vi "Do Something.vi"(8 "error in (no error)":errorcluster, 10 "Bytes to Read":i32, 11 "Inst.MOTOR in":refnum<class "Inst.MOTOR.lvclass">) -> (0 "error out":errorcluster, 3 "Inst.MOTOR out":refnum<class "Inst.MOTOR.lvclass">)   [LabVIEW 2019, in "Inst.MOTOR.lvclass"]
uses:
  Inst.MOTOR.lvclass
  C:/Program Files (x86)/National Instruments/LabVIEW 2019/user.lib/LevyLab/Instrument Framework/SMOs/Instrument/Instrument.lvclass
  Typedefs/Inst.MOTOR.Commands--Enum.ctl
  <userlib>/LevyLab/Instrument Framework/SMOs/Instrument/Instrument.lvclass/Instrument.ctl
  67792bfe-8e2c-4879-abc2-cb448bcec168.vi
  67792bfe-8e2c-4879-abc2-cb448bcec168.vi/e6734212-7c9e-4ce8-a442-683b18d6b7e6.vi
  <userlib>/LevyLab/Instrument Framework/SMOs/Instrument/API/Send and Receive.vi
  67792bfe-8e2c-4879-abc2-cb448bcec168.vi/d08038f8-4acd-46a3-976f-e1cbe8915b66.vi
  <userlib>/LevyLab/Instrument Framework/SMOs/Instrument/Private/Get Client Type.vi
  67792bfe-8e2c-4879-abc2-cb448bcec168.vi/e6734212-7c9e-4ce8-a442-683b18d6b7e6.vi/8ec21fe3-bcb2-49b7-88ee-084ed9ce9051.vi
  67792bfe-8e2c-4879-abc2-cb448bcec168.vi/e6734212-7c9e-4ce8-a442-683b18d6b7e6.vi/b6f90dbd-08b2-43c3-97ed-3e9c828d1fdb.vi
  67792bfe-8e2c-4879-abc2-cb448bcec168.vi/d08038f8-4acd-46a3-976f-e1cbe8915b66.vi/800cf9c4-7383-40cf-9bc6-eb11c7b09f2f.vi
  67792bfe-8e2c-4879-abc2-cb448bcec168.vi/d08038f8-4acd-46a3-976f-e1cbe8915b66.vi/0f5049b1-9107-4d80-b470-81422f3edf74.vi
  67792bfe-8e2c-4879-abc2-cb448bcec168.vi/d08038f8-4acd-46a3-976f-e1cbe8915b66.vi/800cf9c4-7383-40cf-9bc6-eb11c7b09f2f.vi/881d7550-d531-42ab-87b9-010de527541d.vi
  67792bfe-8e2c-4879-abc2-cb448bcec168.vi/d08038f8-4acd-46a3-976f-e1cbe8915b66.vi/800cf9c4-7383-40cf-9bc6-eb11c7b09f2f.vi/262de732-8af3-4438-8d44-96e2fb4cfcee.vi
  <userlib>/LevyLab/Instrument Framework/SMOs/Instrument/Private/Get RC Connection Status.vi
  <userlib>/LevyLab/Instrument Framework/SMOs/Instrument/API/Enum to String.vi
  <userlib>/LevyLab/Instrument Framework/SMOs/RemoteControl/API/Send and Receive.vi
  <vilib>/Utility/Data Type/Get Type Information.vi
  <vilib>/JDP Science/JSONtext/JSON text to Variant.vi
  <userlib>/LevyLab/Instrument Framework/SMOs/Instrument/API/Instrument.GetPublicEvents.vi
  <vilib>/JDP Science/JSONtext/Variant to JSON Text.vi
  <vilib>/National Instruments/GUID Generator/Guid Generator.vi
  <userlib>/LevyLab/Instrument Framework/SMOs/Instrument/API/Instrument.MessageToProcess.vi
  <userlib>/LevyLab/Instrument Framework/SMOs/Instrument/Private/Instrument.MessageFromProcess.EventStructure.vi
  <vilib>/JDP Science/JSONtext/LVClass Serializer/JSONtext LVClass Serializer.lvclass
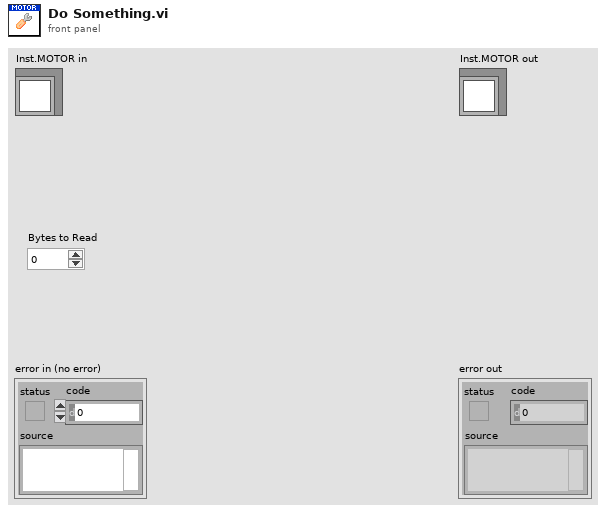
[diagram p1: front panel]
types:
  T1 = typedef "Inst.MOTOR.lvclass/Inst.MOTOR.Commands--Enum.ctl" = enum16{"Encoder Position", "VISA Read", "VISA Write"}
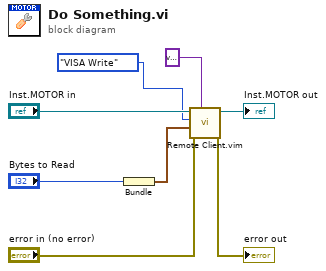
[diagram p0: block diagram]
diagram:
  n1 = Bundle("Bytes to Read"="Bytes to Read") -> (w3:cluster{"Bytes to Read":i32})  [unwired: 1 in]
  n2 = call "Remote Client.vim"("Data Out type"=variant, "error in (no error)"="error in (no error)", "params"=w3, "method"=Inst.MOTOR.Commands--Enum."VISA Write" ("Commands"), "Instrument in"="Inst.MOTOR in") -> ("error out"=→"error out":errorcluster, "Instrument out"=→"Inst.MOTOR out":refnum<class "Inst.MOTOR.lvclass">)  [unwired: 3 in, 2 out]
